vi "Update CPU Bars.vi"(7 "Width":u32, 8 "error in (no error)":errorcluster, 9 "CpuLoadTotal":u32[](array[numeric]), 10 "Array in":refnum<data-value>[](array[refnum]), 11 "Image Editor Handler in":refnum<class "Image Editor Handler.lvclass">) -> (0 "error out":errorcluster, 3 "Editor Handler out":refnum<class "Image Editor Handler.lvclass">)   [LabVIEW 2016]
uses:
  <vilib>/LIEF/Image Editor Handler/Image Editor Handler.lvclass
  <vilib>/LIEF/Forms/Shape/Shape.lvclass
  CPU Bar/CPU Bar.lvclass
  C:/Program Files (x86)/National Instruments/LabVIEW 2016/vi.lib/LIEF/Forms/Shape/Shape.lvclass
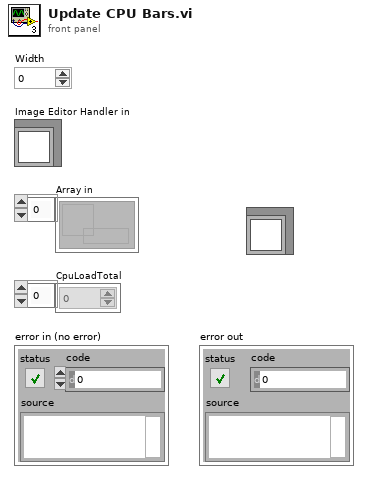
[diagram p1: front panel]
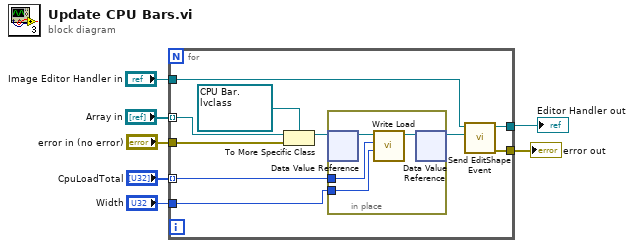
[diagram p0: block diagram]
diagram:
  n1 = for {
    tunnel: "Array in" -> [w15] mode=indexing
    tunnel: "CpuLoadTotal" -> [w13] mode=indexing
    tunnel: "Width" -> [w12]
    tunnel: "Image Editor Handler in" -> [w11]
    tunnel: [w10] -> w1
    tunnel: [w9] -> w6
    tunnel: "error in (no error)" -> [w8]
    n2 = To More Specific Class(target class=refnum<data-value> refnum, reference=w15, error in=w8) -> (specific class reference=w17:refnum<data-value>)  [unwired: 1 out]
    n3 = in-place {
      in-place-border: w13 -> [w19]
      in-place-border: w12 -> [w18]
      n4 = in-place-dvr #1(w17) -> (w20:refnum<class "CPU Bar.lvclass">)  [unwired: 1 out]
      n5 = call "Write Load.vi"("Pic Width"=w18, "CPU Load"=w19, "CPU Bar in"=w20) -> ("CPU Bar out"=w21:refnum<class "CPU Bar.lvclass">)  [unwired: 7 in, 1 out]
      n6 = in-place-dvr #1(w21) -> (w16:refnum<data-value>)  [unwired: 1 out]
    }
    n7 = call <vilib>:"Send EditShape Event.vi"("Shape"=w16, "Editor Handler in"=w11) -> ("error out"=w9:errorcluster, "Editor Handler out"=w10:refnum<class "Image Editor Handler.lvclass">)  [unwired: 8 in]
  }
  "error out" <- w6
  "Editor Handler out" <- w1
